vi "Untitled 412.vi"() -> ()   [LabVIEW 2017]
panel:
  out "standard output 2":string
  out "return code":i32
  out "error out":errorcluster
  out "standard error":string
  out "standard output":string
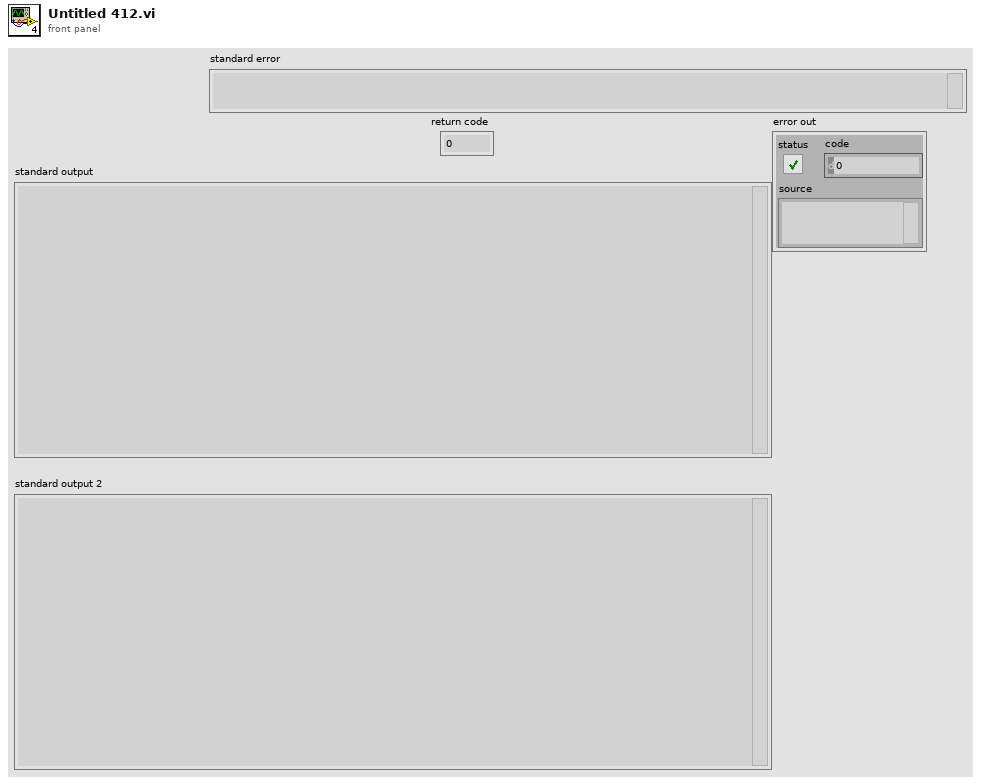
[diagram p1: front panel]
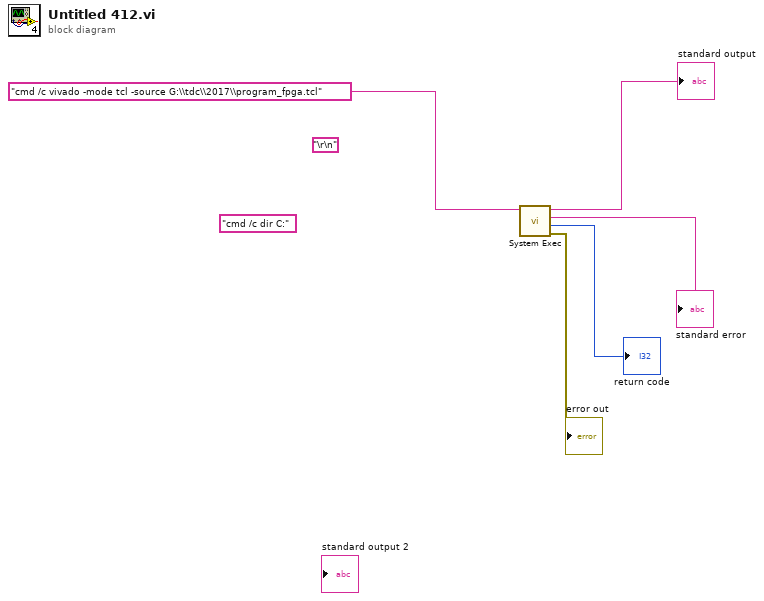
[diagram p0: block diagram]
diagram:
  (unwired) "\r\n"
  (unwired) "cmd /c dir C:" ("command line")
  n1 = call <vilib>:"System Exec.vi"("command line"="cmd /c vivado -mode tcl -source G:\\tdc\\2017\\program_fpga.tcl") -> ("error out"=→"error out":errorcluster, "return code"=→"return code":i32, "standard error"=→"standard error":string, "standard output"=→"standard output":string)  [unwired: 7 in]
